vi "generate_chirp_33120A.vi"() -> ()   [LabVIEW 2014]
panel:
  in  "Hz/step":dbl=-1.0
  in  "Stop Freq (Hz)":dbl=6000.0
  in  "Start Freq (Hz)":dbl=8000.0
  in  "Offset Trim (part per thousand)":i32
  in  "Auto Offset":bool=TRUE
  in  "Manual Offset (V)":dbl=50.0
  in  "Amplitude (V)":dbl=100.0
  in  "Step Length (s)":i32=5
  out "Current Freq":dbl format="%#_13g"
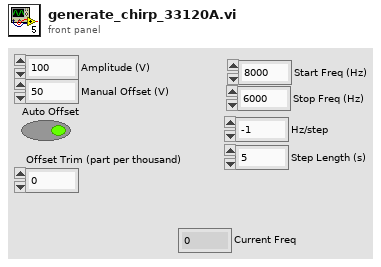
[diagram p1: front panel]
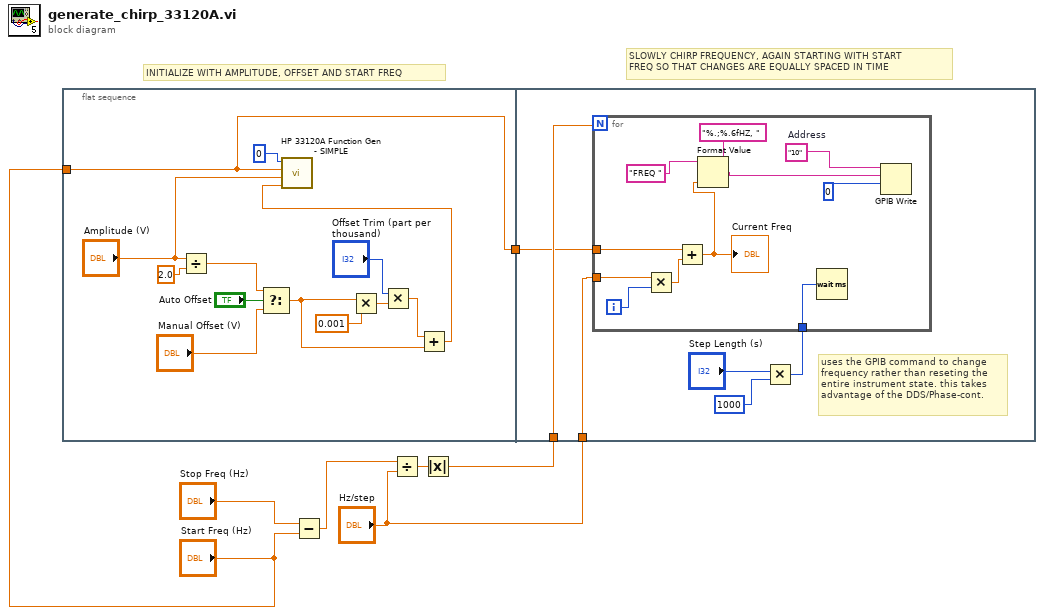
[diagram p0: block diagram]
diagram:
  # "SLOWLY CHIRP FREQUENCY, AGAIN STARTING WITH START\nFREQ SO THAT CHANGES ARE EQUALLY SPACED IN TIME"
  # "INITIALIZE WITH AMPLITUDE, OFFSET AND START FREQ"
  n1 = flat-sequence {
    tunnel: "Start Freq (Hz)" -> [w8]
    tunnel: [w8] -> w1
    tunnel: w3 -> [w23]
    tunnel: "Hz/step" -> [w22]
    tunnel: w1 -> [w21]
    frame #0 {
      n2 = Divide(x="Amplitude (V)", y=2.0) -> (x/y=w18:dbl)
      n3 = Select(t=w18, s="Auto Offset", f="Manual Offset (V)") -> (s? t:f=w16:dbl)
      n4 = Multiply(x=w16, y=0.001) -> (x*y=w13:dbl)
      n5 = Multiply(x="Offset Trim (part per thousand)", y=w13) -> (x*y=w12:dbl)
      n6 = Add(x=w12, y=w16) -> (x+y=w9:dbl)
      n7 = call "HP 33120A Function Gen - SIMPLE.vi"("offset (V)"=w9, "amplitude (V)"="Amplitude (V)", "frequency (Hz)"=w8, "Function Type"=0) -> ()  [unwired: 8 in]
    }
    frame #1 {
      # "uses the GPIB command to change\nfrequency rather than reseting the\nentire instrument state. this takes\nadvantage of the DDS/Phase-cont."
      n8 = Multiply(x="Step Length (s)", y=1000) -> (x*y=w26:i32)
      n9 = for {
        N: w23 -> [_]
        tunnel: w21 -> [w36]
        tunnel: w22 -> [w37]
        tunnel: w26 -> [w33]
        i -> [w34]
        w31 = "10"  # Address
        n10 = Multiply(x=w37, y=w34) -> (x*y=w35:dbl)
        n11 = Add(x=w36, y=w35) -> (x+y=w29:dbl)
        "Current Freq" <- w29
        n12 = Format Value(string ("")="FREQ ", format string="%.;%.6fHZ, ", value (0)=w29) -> (output string=w27:string)
        n13 = Wait (ms)(milliseconds to wait=w33) -> ()  [unwired: 1 out]
        n14 = GPIB Write(0:w31, 1:w27, 2:0) -> ()  [unwired: 1 in, 3 out]
      }
    }
  }
  n15 = Subtract(x="Stop Freq (Hz)", y="Start Freq (Hz)") -> (x-y=w6:dbl)
  n16 = Divide(x=w6, y="Hz/step") -> (x/y=w5:dbl)
  n17 = Absolute Value(x=w5) -> (abs(x)=w3:dbl)
